vi "Menu.vi"() -> ()   [LabVIEW 2016]
uses:
  controls/Enum.ctl
  Course Project/support/Message Queue/Message Cluster.ctl
  <vilib>/FPGAPlugInAG/USB-7856R OEM/niLvFpga_Close_USB-7856R OEM.vi
  <vilib>/FPGAPlugInAG/USB-7856R OEM/niLvFpga_Reset_USB-7856R OEM.vi
  <vilib>/rvi/errors/niLvFpgaAdjustHostInterfaceError.vi
  <vilib>/rvi/interface/nirviCloseFPGA/nirviCloseFPGA.xnode
  controls/FPGAVIreferenceTypeDefScanEngine.ctl
  FPGA Bitfiles/qnmController797_usbRIO_controllerFPGAmu.lvbitx
  controls/FPGAVIreferenceTypeDef.ctl
  <vilib>/rvi/interface/nirviMethod/nirviMethod.xnode
  <vilib>/rvi/interface/nirviReadWriteControl/nirviReadWriteControl.xnode
  Course Project/support/Message Queue/Message Queue.lvlib
  Course Project/support/User Event - Stop/User Event - Stop.lvlib
  <vilib>/Utility/config.llb/NI_LVConfig.lvlib
  <vilib>/Utility/config.llb/Read Key (String).vi
  NiFpgaLv.dll
  controls/EnumSM.ctl
panel:
  in  "Clock":u32=1000000 format="%#_7pHz"
  in  "Custom ADC / DAC":bool
  out "Version":string="Version 02.08.2018"
  in  "Layout":enum32{"1", "2", "3", "4"}(radio)
  in  "Session path":path=path "C:/"
  in  "Create a new module":bool
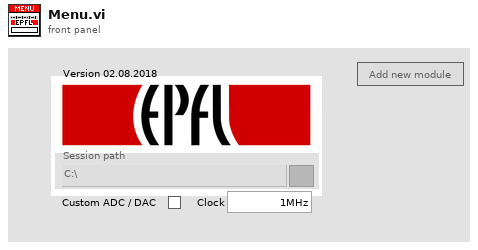
[diagram p1: front panel]
types:
  T1 = typedef "Message Queue.lvlib/All Message Queues.ctl" = cluster{"IU":refnum<queue>}
  T2 = typedef "Enum.ctl" = enum16{"Init", "Read", "Write"}
  T3 = typedef "EnumSM.ctl" = enum16{"Init.Calibrations", "Init.Excitation", "Init.StepMotor", "Init.FeedbackMotion", "Init.Scan", "Init.Signals", "Init.System", "Init.Waveform", "Init.ZController", "Send.Waveform", "Correct.Hysteresis"}
  T4 = enum32{"Bad", "Idle", "Run top level", "Running"}
  T5 = typedef "Message Queue.lvlib/Message Cluster.ctl" = cluster{"Message":string, "Données de message":variant}
  T6 = enum32{"Invalid", "Standard", "Closed", "Hidden", "Minimized", "Maximized"}
  T7 = enum16{"open", "replace", "create", "open or create", "replace or create", "replace or create with confirmation"}
  T8 = typedef "FPGAVIreferenceTypeDef.ctl" = refnum<k20>
  T9 = typedef "FPGAVIreferenceTypeDefScanEngine.ctl" = refnum<k20>
  T10 = typedef "NI_LVConfig.lvlib/Config Data RefNum.ctl" = refnum<k1>
  T11 = enum32{"Invalid", "Standard", "Closed", "Hidden", "Minimized", "Maximized"}[][]
  T12 = cluster{"offset past number":i32, "offset past number":i32}
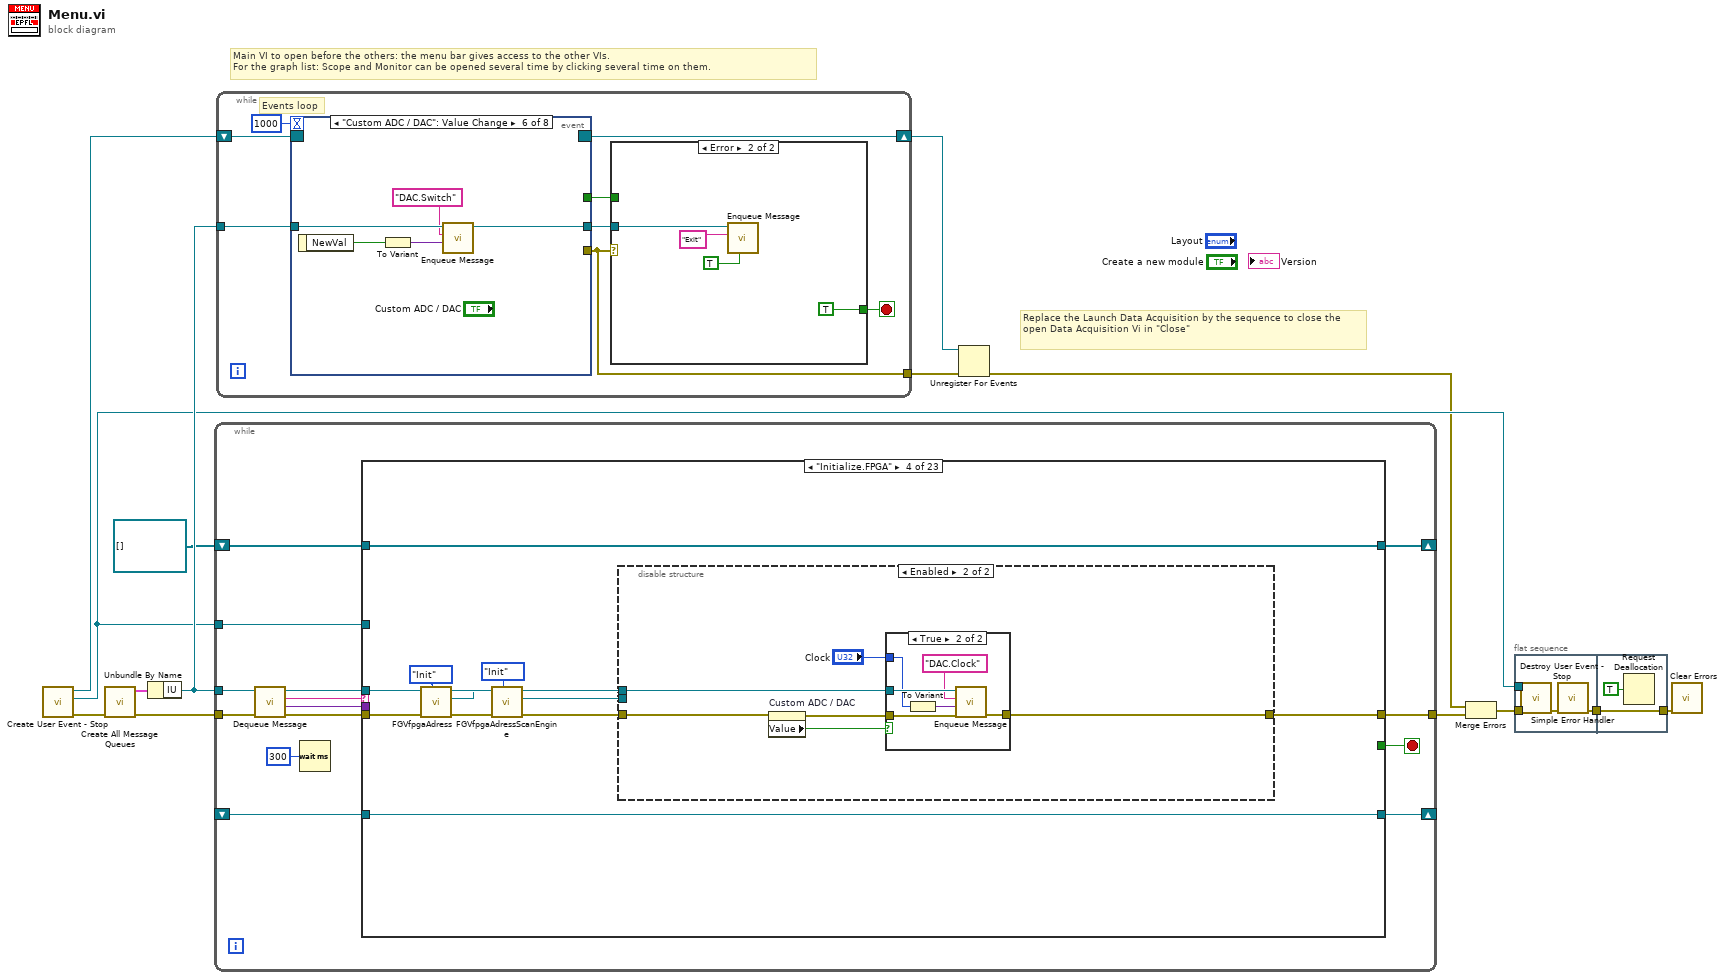
[diagram p0: block diagram]
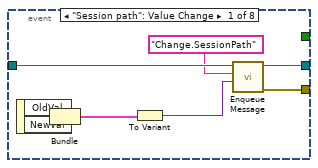
[diagram p3: hidden frame]
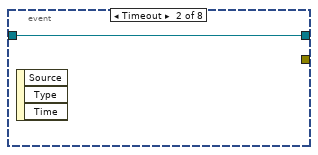
[diagram p4: hidden frame]
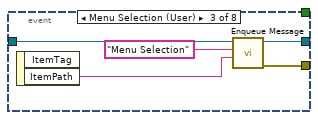
[diagram p5: hidden frame]
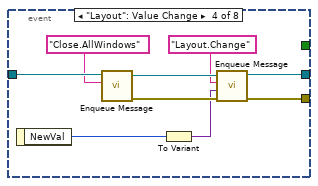
[diagram p6: hidden frame]
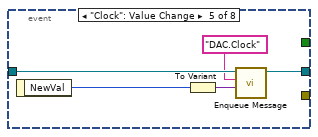
[diagram p7: hidden frame]
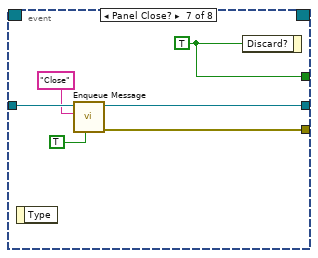
[diagram p8: hidden frame]
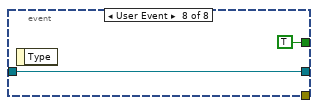
[diagram p9: hidden frame]
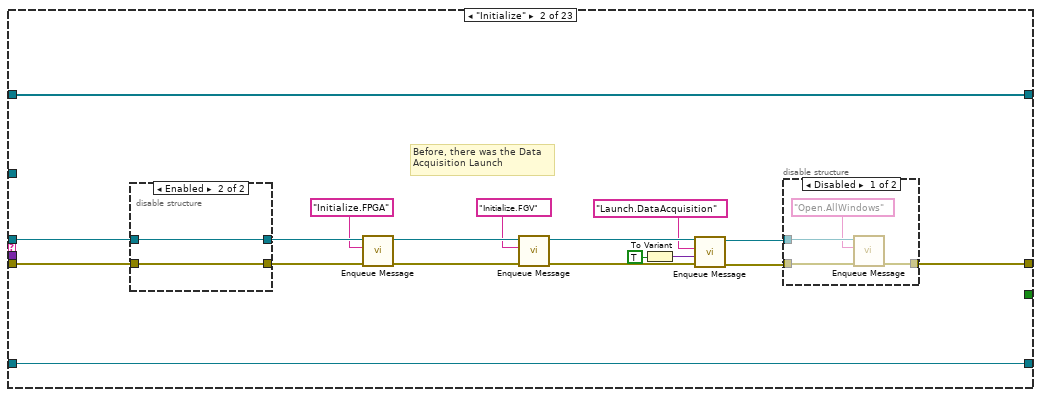
[diagram p11: hidden frame]
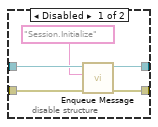
[diagram p12: hidden frame]
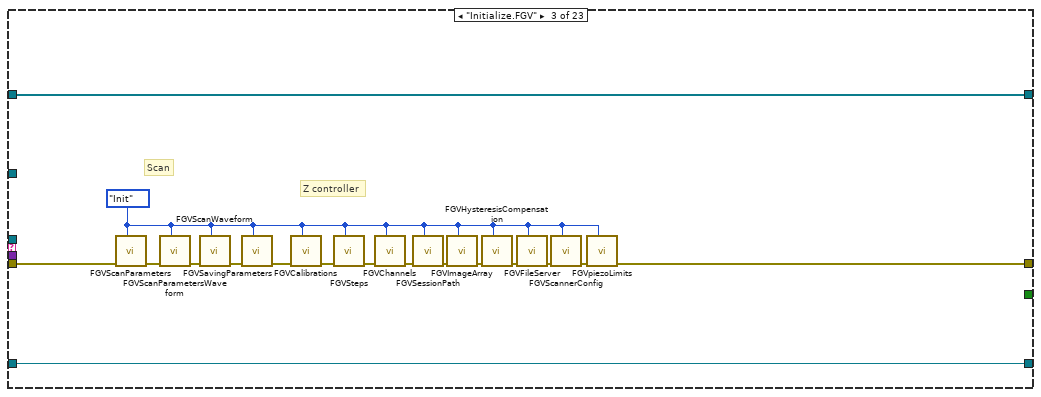
[diagram p14: hidden frame]
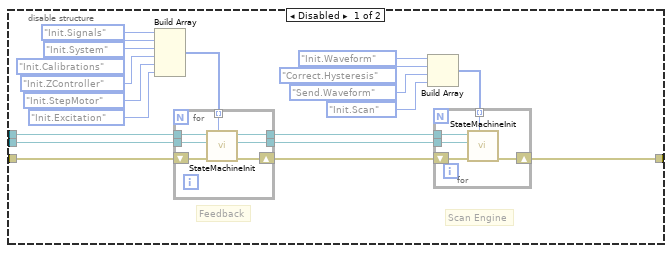
[diagram p15: hidden frame]
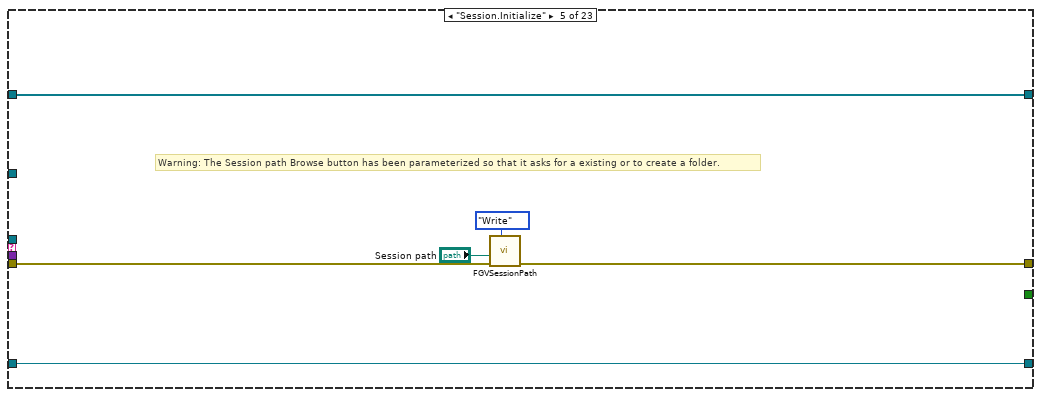
[diagram p17: hidden frame]
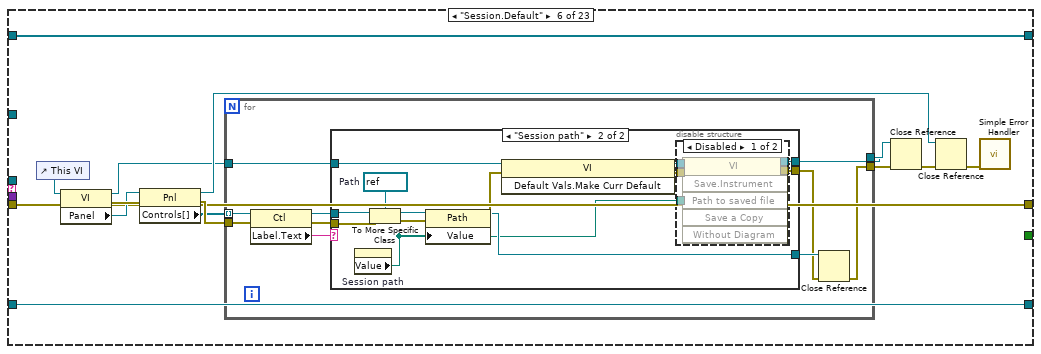
[diagram p18: hidden frame]
diagram:
  # "Main VI to open before the others: the menu bar gives access to the other VIs.\nFor the graph list: Scope and Monitor can be opened several time by clicking several time on them."
  # "Replace the Launch Data Acquisition by the sequence to close the open Data Acquisition Vi in \"Close\""
  n1 = call "Create User Event - Stop.vi"() -> ("sortie d'erreur"=w9:errorcluster, "Événement utilisateur - Arrêt"=w7:refnum<user-event>, "Refnum Enregistrement à l'événement Arrêt"=w10:refnum<event-registration>)  [unwired: 9 in]
  n2 = call "Create All Message Queues.vi"("ErrorIn"=w9) -> ("ErrorOut"=w14:errorcluster, "MessageQueueOut"=w13:T1)  [unwired: 9 in]
  n3 = Unbundle By Name(w13) -> ("IU"=w11:refnum<queue>)
  n4 = while {
    tunnel: w11 -> [w20]
    tunnel: w7 -> [w26]
    tunnel: w14 -> [w25]
    tunnel: [w27] -> w12
    shift-right: [w18] -> _
    shift-left: refnum<vi>[] [] -> [w17]
    shift-right: [w16] -> _
    shift-left: _ -> [w15]
    stop <- w28 stop-if-true
    n5 = call "Dequeue Message.vi"("entrée d'erreur (pas d'erreur)"=w25, "File d'attente de messages"=w20) -> ("sortie d'erreur"=w24:errorcluster, "Données de message"=w22:variant, "Message"=w23:string, "File d'attente de message dup."=w21:refnum<queue>)  [unwired: 6 in]
    n6 = Wait (ms)(milliseconds to wait=u32 300) -> ()  [unwired: 1 out]
    n7 = case "Conditions des messages" shown="\"Initialize.FPGA\"" w23 {
      selector: w23 -> [_ _ _ _ _ _ _ _ _ _ _ _ _ _ _ _ _ _ _ _ _ _ w637]
      tunnel: w21 -> [_ w47 _ w89 _ _ _ _ _ _ _ _ _ _ _ _ _ _ w544 w565 _ w623 _]
      tunnel: w24 -> [w31 w41 w70 w88 w136 w140 w192 w196 w248 w285 w311 w317 w378 w387 w393 w413 w436 w477 w542 w554 w580 w620 _]
      tunnel: [w31 w46 w63 w83 w135 w140 w192 w197 w252 w283 w311 w320 w377 w387 w390 errorcluster {"status"=FALSE, "code"=0, "source"=""} ("error out") w437 w473 w529 w555 w577 w601 w635] -> w27
      tunnel: [_ _ _ _ _ _ _ _ _ _ _ _ _ _ _ _ _ _ _ _ _ TRUE _] -> w28
      tunnel: w22 -> [_ _ _ _ _ _ _ w195 w246 w284 _ _ _ _ _ w412 w434 w476 w541 _ _ _ _]
      tunnel: w26 -> [_ _ _ _ _ _ _ _ _ _ _ _ _ _ _ _ _ _ _ _ _ w619 _]
      tunnel: [w30 w44 w78 w87 w139 w141 w189 w207 w254 w287 w309 w315 refnum<vi>[] [] w386 w391 w404 w431 w465 w531 w558 w594 w617 w633] -> w18
      tunnel: w17 -> [w30 w44 w78 w87 w139 w141 w189 w207 w254 w287 w309 _ w376 w386 w392 w404 w431 w465 w531 w558 w594 w617 w633]
      tunnel: [w29 w43 w77 w86 w138 w142 w187 w206 w253 w286 w310 w312 w374 w385 w389 w403 w430 w464 w530 w557 w593 w616 w632] -> w16
      tunnel: w15 -> [w29 w43 w77 w86 w138 w142 _ w206 w253 w286 w310 w314 w374 w385 w389 w403 w430 w464 w530 w557 w593 w616 w632]
      frame " ------- Init -------" {
      }
      frame "Initialize" {
        # "Before, there was the Data \nAcquisition Launch"
        n8 = disable-structure shown="Enabled" {
          disable-tunnel: [w54 w56] -> w48
          disable-tunnel: w47 -> [w53 w56]
          disable-tunnel: [w51 w55] -> w42
          disable-tunnel: w41 -> [w50 w55]
          frame Disabled {
            n9 = call "Enqueue Message.vi"("error in"=w50, "Message"="Session.Initialize", "Queue"=w53) -> ("error out"=w51:errorcluster, "Queue dup."=w54:refnum<queue>)  [unwired: 7 in]
          }
          frame Enabled {
          }
        }
        n10 = call "Enqueue Message.vi"("error in"=w42, "Message"="Initialize.FPGA", "Queue"=w48) -> ("error out"=w39:errorcluster, "Queue dup."=w40:refnum<queue>)  [unwired: 7 in]
        n11 = call "Enqueue Message.vi"("error in"=w39, "Message"="Initialize.FGV", "Queue"=w40) -> ("error out"=w35:errorcluster, "Queue dup."=w49:refnum<queue>)  [unwired: 7 in]
        n12 = To Variant(anything=TRUE) -> (Variant=w32:variant)
        n13 = call "Enqueue Message.vi"("error in"=w35, "Data"=w32, "Message"="Launch.DataAcquisition", "Queue"=w49) -> ("error out"=w36:errorcluster, "Queue dup."=w34:refnum<queue>)  [unwired: 6 in]
        n14 = disable-structure shown="Disabled" {
          disable-tunnel: w34 -> [w60 _]
          disable-tunnel: [w59 w61] -> w46
          disable-tunnel: w36 -> [w57 w61]
          frame Disabled {
            n15 = call "Enqueue Message.vi"("error in"=w57, "Message"="Open.AllWindows", "Queue"=w60) -> ("error out"=w59:errorcluster)  [unwired: 7 in, 1 out]
          }
          frame Enabled {
          }
        }
      }
      frame "Initialize.FGV" {
        w62 = Enum."Init" ("Enum")
        # "Z controller"
        # "Scan"
        n16 = call "FGVScanParameters.vi"("Enum"=w62, "error in"=w70) -> ("error out"=w76:errorcluster)  [unwired: 8 in, 1 out]
        n17 = call "FGVScanParametersWaveform.vi"("Enum"=w62, "error in"=w76) -> ("error out"=w75:errorcluster)  [unwired: 8 in, 1 out]
        n18 = call "FGVScanWaveform.vi"("Enum"=w62, "error in"=w75) -> ("error out"=w74:errorcluster)  [unwired: 8 in, 1 out]
        n19 = call "FGVSavingParameters.vi"("Enum"=w62, "error in"=w74) -> ("error out"=w73:errorcluster)  [unwired: 6 in, 3 out]
        n20 = call "FGVCalibrations.vi"("Enum"=w62, "error in"=w73) -> ("error out"=w72:errorcluster)  [unwired: 8 in, 1 out]
        n21 = call "FGVSteps.vi"("Enum"=w62, "error in"=w72) -> ("error out"=w71:errorcluster)  [unwired: 6 in, 3 out]
        n22 = call "FGVChannels.vi"("Enum"=w62, "error in"=w71) -> ("error out"=w69:errorcluster)  [unwired: 5 in, 4 out]
        n23 = call "FGVSessionPath.vi"("Enum"=w62, "error in"=w69) -> ("error out"=w68:errorcluster)  [unwired: 8 in, 1 out]
        n24 = call "FGVImageArray.vi"("Enum"=w62, "error in"=w68) -> ("error out"=w67:errorcluster)  [unwired: 8 in, 1 out]
        n25 = call "FGVHysteresisCompensation.vi"("Enum"=w62, "error in"=w67) -> ("error out"=w66:errorcluster)  [unwired: 7 in, 2 out]
        n26 = call "FGVFileServer.vi"("Enum"=w62, "error in"=w66) -> ("error out"=w65:errorcluster)  [unwired: 8 in, 1 out]
        n27 = call "FGVScannerConfig.vi"("Enum"=w62, "error in"=w65) -> ("error out"=w64:errorcluster)  [unwired: 7 in, 2 out]
        n28 = call "FGVpiezoLimits.vi"("Enum"=w62, "error in"=w64) -> ("error out"=w63:errorcluster)  [unwired: 8 in, 1 out]
      }
      frame "Initialize.FPGA" {
        n29 = call "FGVfpgaAdress.vi"("Enum"=Enum."Init", "error in"=w88) -> ("error out"=w80:errorcluster, "FPGA VI Reference Out"=w84:T8)  [unwired: 4 in, 4 out]
        n30 = call "FGVfpgaAdressScanEngine.vi"("Enum"=Enum."Init", "error in"=w80) -> ("error out"=w85:errorcluster, "FPGA.SEout"=w82:T9)  [unwired: 5 in, 3 out]
        n31 = disable-structure shown="Enabled" {
          disable-tunnel: w85 -> [w108 w126]
          disable-tunnel: w84 -> [w107 _]
          disable-tunnel: [w104 w124] -> w83
          disable-tunnel: w82 -> [w95 _]
          disable-tunnel: w89 -> [_ w122]
          frame Disabled {
            # "Feedback"
            # "Scan Engine"
            n32 = Build Array(EnumSM."Init.Signals" ("Enum"), EnumSM."Init.System" ("Enum"), EnumSM."Init.Calibrations" ("Enum"), EnumSM."Init.ZController" ("Enum"), EnumSM."Init.StepMotor" ("Enum"), EnumSM."Init.Excitation" ("Enum")) -> (w93:T3[])
            n33 = for {
              tunnel: w95 -> [w111]
              shift-right: [w112] -> w105
              shift-left: w108 -> [w115]
              tunnel: w93 -> [w110] mode=indexing
              tunnel: [w109] -> w92
              tunnel: w107 -> [w114]
              tunnel: [w113] -> w106
              n34 = call "StateMachineInit.vi"("Enum"=w110, "Error In"=w115, "FPGA.SEin"=w111, "FPGA.FBin"=w114) -> ("error out"=w112:errorcluster, "FPGA.SEout"=w109:T9, "FPGA.FBout"=w113:T8)  [unwired: 5 in]
            }
            n35 = Build Array(EnumSM."Init.Waveform" ("Enum"), EnumSM."Correct.Hysteresis" ("Enum"), EnumSM."Send.Waveform" ("Enum"), EnumSM."Init.Scan" ("Enum")) -> (w94:T3[])
            n36 = for {
              tunnel: w106 -> [w120]
              shift-right: [w118] -> w104
              shift-left: w105 -> [w119]
              tunnel: w94 -> [w117] mode=indexing
              tunnel: w92 -> [w116]
              n37 = call "StateMachineInit.vi"("Enum"=w117, "Error In"=w119, "FPGA.SEin"=w116, "FPGA.FBin"=w120) -> ("error out"=w118:errorcluster)  [unwired: 5 in, 2 out]
            }
          }
          frame Enabled {
            n38 = property on="Custom ADC / DAC" class="Bool (strict)"(error in=w126) -> (error out=w123:errorcluster, "Value"=w125:bool)  [unwired: 1 in, 1 out]
            n39 = case shown="True" w125 {
              tunnel: w122 -> [_ w133]
              tunnel: "Clock" -> [_ w132]
              tunnel: [w127 w129] -> w124
              tunnel: w123 -> [w127 w128]
              frame False {
              }
              frame True {
                n40 = To Variant(anything=w132) -> (Variant=w130:variant)
                n41 = call "Enqueue Message.vi"("error in"=w128, "Data"=w130, "Message"="DAC.Clock", "Queue"=w133) -> ("error out"=w129:errorcluster)  [unwired: 6 in, 1 out]
              }
            }
          }
        }
      }
      frame "Session.Initialize" {
        # "Warning: The Session path Browse button has been parameterized so that it asks for a existing or to create a folder."
        n42 = call "FGVSessionPath.vi"("Enum"=Enum."Write", "error in"=w136, "sessionPathIn"="Session path") -> ("error out"=w135:errorcluster)  [unwired: 7 in, 1 out]
      }
      frame "Session.Default" {
        n43 = control-ref of="This VI"() -> (w143:refnum<vi>)
        n44 = property on="Property Node" class="VI"(reference=w143) -> (reference out=w146:refnum<vi>, error out=w147:errorcluster, "Panel"=w144:refnum<vi>)  [unwired: 1 in]
        n45 = property on="Property Node" class="Pnl"(reference=w144, error in=w147) -> (reference out=w153:refnum<vi>, error out=w148:errorcluster, "Controls[]"=w145:refnum<vi>[])
        n46 = for {
          tunnel: w145 -> [w162] mode=indexing
          tunnel: w146 -> [w163]
          tunnel: w148 -> [w159]
          tunnel: [w154] -> w149
          tunnel: [w157] -> w150
          n47 = property on="Property Node" class="Ctl"(reference=w162, error in=w159) -> (reference out=w160:refnum<vi>, error out=w158:errorcluster, "Label.Text"=w161:string)
          n48 = case shown="\"Session path\"" w161 {
            tunnel: w163 -> [w165 w179]
            tunnel: w160 -> [w164 w174]
            tunnel: w158 -> [w166 w173]
            tunnel: [w166 w171] -> w155
            tunnel: [w165 w170] -> w157
            tunnel: [w164 w168] -> w156
            frame Default {
            }
            frame "Session path" {
              w176 = refnum<vi> refnum  # Path
              n49 = property on="Session path" class="Path"() -> ("Value"=w167:path)  [unwired: 2 in, 2 out]
              n50 = To More Specific Class(target class=w176, reference=w174, error in=w173) -> (specific class reference=w175:refnum<vi>, error out=w172:errorcluster)
              n51 = property on="Property Node" class="Path"(reference=w175, error in=w172, "Value"=w167) -> (reference out=w168:refnum<vi>, error out=w169:errorcluster)
              n52 = invoke class="VI" method="Default Vals.Make Curr Default"(reference=w179, error in=w169) -> (reference out=w178:refnum<vi>, error out=w177:errorcluster)  [unwired: 1 in, 1 out]
              n53 = disable-structure shown="Disabled" {
                disable-tunnel: w178 -> [w184 w186]
                disable-tunnel: w177 -> [w183 w185]
                disable-tunnel: [w182 w185] -> w171
                disable-tunnel: [w181 w186] -> w170
                disable-tunnel: w167 -> [w180 _]
                frame Disabled {
                  n54 = invoke class="VI" method="Save.Instrument"(reference=w184, error in=w183, "Path to saved file"=w180) -> (reference out=w181:refnum<vi>, error out=w182:errorcluster)  [unwired: 3 in, 4 out]
                }
                frame Enabled {
                }
              }
            }
          }
          n55 = Close Reference(reference=w156, error in (no error)=w155) -> (error out=w154:errorcluster)
        }
        n56 = Close Reference(reference=w150, error in (no error)=w149) -> (error out=w152:errorcluster)
        n57 = Close Reference(reference=w153, error in (no error)=w152) -> (error out=w151:errorcluster)
        n58 = call <vilib>:"Simple Error Handler.vi"("error in (no error)"=w151) -> ()  [unwired: 4 in, 5 out]
      }
      frame "Load.ConfigurationFile" {
        n59 = local read "Session path"() -> (w190:path)
        n60 = Build Path(base path=w190, name or relative path=path "ConfigurationFile.ini" ("default name")) -> (appended path=w188:path)
        n61 = call <vilib>:"Open Config Data.vi"("configuration file path"=w188) -> ("refnum"=w187:T10)  [unwired: 2 in, 8 out]
      }
      frame "Launch.DataAcquisition" {
        n62 = Variant To Data(error in=w196, type=TRUE, Variant=w195) -> (data=w205:bool, error out=w193:errorcluster)
        n63 = call <vilib>:"Application Directory.vi"() -> ("Application Directory"=w202:path)
        n64 = Build Path(base path=w202, name or relative path="FrontPanel\\subVIs\\DataAcquisition.vi") -> (appended path=w201:path)
        n65 = Open VI Reference(vi path=w201, error in (no error)=w193) -> (vi reference=w204:refnum<vi>, error out=w200:errorcluster)  [unwired: 4 in]
        n66 = case "Check the state of the VI: running or closed" shown="True" w205 {
          tunnel: w200 -> [w218 w228]
          tunnel: w204 -> [w211 w236]
          tunnel: [w208 w226] -> w198
          frame False {
            n67 = property class="VI"(reference=w211) -> (reference out=w219:refnum<vi>, "Exec.State"=w213:T4)  [unwired: 1 in, 1 out]
            n68 = Equal?(x=T4."Bad" ("Execution:State"), y=w213) -> (x = y?=w215:bool)
            n69 = Equal?(x=w213, y=T4."Idle" ("Execution:State")) -> (x = y?=w216:bool)
            n70 = Or(x=w215, y=w216) -> (x .or. y?=w217:bool)
            n71 = case shown="False" w217 {
              tunnel: [w223 w225] -> w210
              tunnel: [w222 w224] -> w209
              tunnel: w218 -> [w221 w224]
              tunnel: w219 -> [w220 w225]
              frame False {
                n72 = invoke class="VI" method="Abort VI"(reference=w220, error in=w221) -> (reference out=w223:refnum<vi>, error out=w222:errorcluster)  [unwired: 1 in, 1 out]
              }
              frame True {
              }
            }
            n73 = Close Reference(reference=w210, error in (no error)=w209) -> (error out=w208:errorcluster)
          }
          frame True {
            n74 = property class="VI"(reference=w236, error in=w228) -> (reference out=w235:refnum<vi>, error out=w227:errorcluster, "Exec.State"=w233:T4)
            n75 = Equal?(x=T4."Run top level" ("Execution:State"), y=w233) -> (x = y?=w231:bool)
            n76 = Equal?(x=w233, y=T4."Running" ("Execution:State")) -> (x = y?=w230:bool)
            n77 = Or(x=w231, y=w230) -> (x .or. y?=w229:bool)
            n78 = case shown="False" w229 {
              tunnel: [w238 w243] -> _
              tunnel: [w237 w242] -> w226
              tunnel: w227 -> [w239 w242]
              tunnel: w235 -> [w240 w243]
              frame False {
                n79 = invoke class="VI" method="Run VI"(reference=w240, error in=w239, "Wait until done"=FALSE ("Wait Until Done")) -> (reference out=w238:refnum<vi>, error out=w237:errorcluster)  [unwired: 2 in, 3 out]
              }
              frame True {
              }
            }
          }
        }
        n80 = call "FGVImageArray.vi"("Enum"=Enum."Init", "error in"=w198) -> ("error out"=w197:errorcluster)  [unwired: 8 in, 1 out]
      }
      frame "DAC.Switch" {
        n81 = Variant To Data(error in=w248, type=TRUE, Variant=w246) -> (data=w244:bool, error out=w247:errorcluster)
        n82 = call "FGVfpgaAdress.vi"("Enum"=Enum."Read", "error in"=w247) -> ("error out"=w250:errorcluster, "FPGA VI Reference Out"=w249:T8)  [unwired: 4 in, 4 out]
        n83 = xnode "Read/Write Control"("FPGA VI Reference In"=w249, "error in"=w250, "aio.o.fastInput"=w244) -> ("error out"=w252:errorcluster)  [unwired: 1 out]
      }
      frame "DAC.Clock" {
        w260 = 2.0 ("y")
        # "4 for 80MHz\n1 for 1Mhz"
        # "2 for the usb rio"
        n84 = Variant To Data(error in=w285, type=u32 0 ("NewVal"), Variant=w284) -> (data=w278:u32, error out=w288:errorcluster)
        n85 = call "FGVfpgaAdress.vi"("Enum"=Enum."Read", "error in"=w288) -> ("error out"=w276:errorcluster, "baseClockOut"=w256:u32, "FPGA VI Reference Out"=w273:T8, "voltageRange(+/-)Out"=w274:dbl)  [unwired: 4 in, 2 out]
        n86 = Multiply(x=w256, y=u32 1 ("x")) -> (x*y=w257:u32)
        n87 = Divide(x=w257, y=w278) -> (x/y=w272:dbl)
        n88 = Divide(x=w272, y=w260) -> (x/y=w269:dbl)
        n89 = To Unsigned Word Integer(number=w269) -> (unsigned 16bit integer=w261:u16)
        n90 = xnode "Read/Write Control"("FPGA VI Reference In"=w273, "error in"=w276, "aio.p.fastADCclockdec"=w261) -> ("FPGA VI Reference Out"=w271:T8, "error out"=w277:errorcluster)
        n91 = Divide(x=w257, y=w261) -> (x/y=w259:dbl)
        n92 = Divide(x=w259, y=w260) -> (x/y=w258:dbl)
        n93 = To Unsigned Long Integer(number=w258) -> (unsigned 32bit integer=w264:u32)
        n94 = call "FGVfpgaAdress.vi"("ioFreqHzIn"=w264, "Enum"=Enum."Write", "error in"=w277, "BaseClockIn"=w256, "FPGA VI Reference In"=w271, "voltageRange(+/-)In"=w274) -> ("error out"=w263:errorcluster)  [unwired: 5 out]
        n95 = property on="Clock" class="DigNum (strict)"(error in=w263, "Value"=w264) -> (error out=w262:errorcluster)  [unwired: 1 in, 1 out]
        n96 = call "IsVIRunning.vi"("error in (no error)"=w262, "name or relative path"="FrontPanel\\Excitation.vi") -> ("error out"=w267:errorcluster, "RunningVI?"=w266:bool)  [unwired: 8 in]
        n97 = disable-structure shown="Enabled" {
          disable-tunnel: [w291 w300] -> w268
          disable-tunnel: w267 -> [w290 w300]
          disable-tunnel: w266 -> [w289 _]
          frame Enabled {
            n98 = case shown="True" w289 {
              tunnel: [w292 w298] -> w291
              tunnel: w290 -> [w292 w294]
              frame False {
              }
              frame True {
                n99 = Obtain Queue(name (unnamed)="Excitation" ("QueueName"), element data type=T5 {"Message"="", "Données de message"=variant} ("Cluster Message"), error in (no error)=w294) -> (queue out=w299:refnum<queue>, error out=w293:errorcluster)  [unwired: 2 in, 1 out]
                n100 = call "Enqueue Message.vi"("error in"=w293, "Message"="Menu.ChangeClock", "Queue"=w299) -> ("error out"=w298:errorcluster)  [unwired: 7 in, 1 out]
              }
            }
          }
          frame Disabled {
          }
        }
        n101 = call "IsVIRunning.vi"("error in (no error)"=w268, "name or relative path"="FrontPanel\\ZController.vi") -> ("error out"=w281:errorcluster, "RunningVI?"=w280:bool)  [unwired: 8 in]
        n102 = case shown="True" w280 {
          tunnel: [w301 w307] -> w283
          tunnel: w281 -> [w301 w303]
          frame False {
          }
          frame True {
            n103 = Obtain Queue(name (unnamed)="ZController" ("QueueName"), element data type=T5 {"Message"="", "Données de message"=variant} ("Cluster Message"), error in (no error)=w303) -> (queue out=w308:refnum<queue>, error out=w302:errorcluster)  [unwired: 2 in, 1 out]
            n104 = call "Enqueue Message.vi"("error in"=w302, "Message"="Controllers.IOFrequency", "Queue"=w308) -> ("error out"=w307:errorcluster)  [unwired: 7 in, 1 out]
          }
        }
      }
      frame "------- Windows -------" {
      }
      frame "Open.AllWindows" {
        w313 = "WindowPositions"  # Section
        w316 = T11 [[enum."Standard", enum."Standard", enum."Standard", enum."Standard"], [enum."Standard", enum."Standard", enum."Hidden", enum."Standard"], [enum."Standard", enum."Standard", enum."Standard", enum."Standard"], [enum."Standard", enum."Standard", enum."Hidden", enum."Standard"], [enum."Standard", enum."Hidden", enum."Standard", enum."Hidden"], [enum."Closed", enum."Standard", enum."Standard", enum."Hidden"], [enum."Closed", enum."Hidden", enum."Standard", enum."Standard"], [enum."Closed", enum."Closed", enum."Closed", enum."Closed"]] items=["Invalid", "Standard", "Closed", "Hidden", "Minimized", "Maximized"]
        # "Take the names from the menu.rtm"
        # "Add window position from configuration file"
        # "4"
        # "3"
        # "2"
        # "Layout"
        # "1"
        # "Windows config for layouts"
        n105 = for {
          tunnel: "Monitor" -> [w343]
          tunnel: string[] ["Calibration", "Signals", "Scan", "ZController", "Monitor", "3xMonitor", "4xMonitor", "Waveforms"] -> [w327] mode=indexing
          tunnel: w316 -> [w334]
          tunnel: w317 -> [_]
          tunnel: [w330] -> w320
          tunnel: [w329] -> w315 mode=indexing
          tunnel: w314 -> [w324]
          tunnel: w313 -> [w323]
          tunnel: [w322] -> w312
          i -> [w333]
          n106 = Not Equal?(x=w327, y=w343) -> (x != y?=w335:bool)
          n107 = Select(t=".vi", s=w335, f=".vit") -> (s? t:f=w326:string)
          n108 = local read "Layout"() -> (w332:enum32{"1", "2", "3", "4"})
          n109 = call <vilib>:"Application Directory.vi"() -> ("Application Directory"=w339:path)
          n110 = Concatenate Strings("FrontPanel\\" ("string"), w327, w326) -> (w342:string)
          n111 = Concatenate Strings(w327, w326) -> (w325:string)
          n112 = Build Path(base path=w339, name or relative path=w342) -> (appended path=w341:path)
          n113 = Index Array(array=w334, index (row)=w333, index (col)=w332) -> (element=w331:T6)
          n114 = Open VI Reference(vi path=w341) -> (vi reference=w338:refnum<vi>, error out=w321:errorcluster)  [unwired: 5 in]
          n115 = case shown="No Error" w321 {
            selector: w321 -> [w344 w357]
            tunnel: w338 -> [w353 w358]
            tunnel: w331 -> [w352 _]
            tunnel: [w351 w357] -> w330
            tunnel: [w350 w358] -> w329
            tunnel: [w349 _] -> w328
            frame No Error {
              n116 = invoke class="VI" method="FP.Open"(reference=w353, error in=w344, "Activate"=TRUE ("Activate?"), "State"=w352) -> (reference out=w348:refnum<vi>, error out=w347:errorcluster)  [unwired: 1 in, 3 out]
              n117 = property class="VI"(reference=w348, error in=w347) -> (reference out=w346:refnum<vi>, error out=w345:errorcluster, "Panel"=w349:refnum<vi>)
              n118 = invoke class="VI" method="Run VI"(reference=w346, error in=w345, "Wait until done"=FALSE ("Wait Until Done"), "Auto Dispose Ref"=FALSE ("Auto Dispose Reference")) -> (reference out=w350:refnum<vi>, error out=w351:errorcluster)  [unwired: 1 in, 3 out]
            }
            frame Error {
            }
          }
          n119 = disable-structure shown="Disabled" {
            disable-tunnel: w328 -> [w372 _]
            disable-tunnel: w325 -> [w370 _]
            disable-tunnel: w324 -> [w369 w373]
            disable-tunnel: w323 -> [w368 _]
            disable-tunnel: [w367 w373] -> w322
            frame Disabled {
              n120 = call-poly <vilib>:"Read Key.vi"("section"=w368, "key"=w370, "refnum"=w369) -> ("value"=w366:string, "refnum out"=w367:T10)  [unwired: 5 in, 2 out]
              n121 = call <vilib>:"Space Constant.vi"() -> ("String"=w365:string)
              n122 = Match Pattern(string=w366, regular expression=w365) -> (before substring=w363:string, after substring=w362:string)  [unwired: 1 in, 2 out]
              n123 = call <vilib>:"Space Constant.vi"() -> ("String"=w364:string)
              n124 = Match Pattern(string=w362, regular expression=w364) -> (before substring=w359:string)  [unwired: 1 in, 3 out]
              n125 = Decimal String To Number(string=w363) -> (offset past number=w361:i32)  [unwired: 2 in, 1 out]
              n126 = Decimal String To Number(string=w359) -> (offset past number=w360:i32)  [unwired: 2 in, 1 out]
              n127 = Bundle("offset past number"=w361, "offset past number"=w360) -> (w371:T12)  [unwired: 1 in]
              n128 = property class="Pnl"(reference=w372, "Position"=w371) -> ()  [unwired: 1 in, 2 out]
            }
            frame Enabled {
            }
          }
        }
      }
      frame "Close.AllWindows" {
        n129 = for {
          tunnel: w378 -> [w380]
          tunnel: [w384] -> w377
          tunnel: w376 -> [w381] mode=indexing
          n130 = property class="VI"(reference=w381, error in=w380, "Front Panel Window:State"=T6."Closed") -> (reference out=w383:refnum<vi>, error out=w382:errorcluster)
          n131 = Close Reference(reference=w383, error in (no error)=w382) -> (error out=w384:errorcluster)
        }
      }
      frame "------- Layouts -------" {
      }
      frame "Layout.Change" {
        w394 = T11 [[enum."Standard", enum."Standard", enum."Standard", enum."Standard"], [enum."Standard", enum."Standard", enum."Hidden", enum."Hidden"], [enum."Hidden", enum."Hidden", enum."Standard", enum."Hidden"], [enum."Hidden", enum."Hidden", enum."Hidden", enum."Standard"], [enum."Closed", enum."Closed", enum."Closed", enum."Closed"], [enum."Closed", enum."Closed", enum."Closed", enum."Closed"], [enum."Closed", enum."Closed", enum."Closed", enum."Closed"], [enum."Closed", enum."Closed", enum."Closed", enum."Closed"]] items=["Invalid", "Standard", "Closed", "Hidden", "Minimized", "Maximized"]
        n132 = local read "Layout"() -> (w388:enum32{"1", "2", "3", "4"})
        n133 = for {
          tunnel: w394 -> [w402]
          tunnel: w393 -> [w400]
          tunnel: w392 -> [w398] mode=indexing
          tunnel: [w397] -> w391 mode=indexing
          tunnel: [w396] -> w390
          tunnel: w388 -> [w395]
          i -> [w401]
          n134 = Index Array(array=w402, index (row)=w401, index (col)=w395) -> (element=w399:T6)
          n135 = property class="VI"(reference=w398, error in=w400, "Front Panel Window:State"=w399) -> (reference out=w397:refnum<vi>, error out=w396:errorcluster)
        }
      }
      frame "Open Settings" {
        # "Replace when there will finally be a Settings.ini file"
        n136 = Variant To Data(error in=w413, type=path "", Variant=w412) -> (data=w407:path, error out=w410:errorcluster)
        n137 = call "FGVSessionPath.vi"("Enum"=Enum."Write", "error in"=w410, "sessionPathIn"=w407) -> ("error out"=w409:errorcluster, "sessionPathOut"=w406:path)  [unwired: 7 in]
        n138 = disable-structure shown="Disabled" {
          disable-tunnel: w409 -> [w416 _]
          disable-tunnel: w406 -> [w414 _]
          frame Disabled {
            (unwired) "Session.ini"
            # "Do the same for Session"
            n139 = Build Path(base path=w414, name or relative path="Settings.ini") -> (appended path=w422:path)
            n140 = Open/Create/Replace File(file path (use dialog)=w422, error in=w416, operation (0:open)=T7."replace or create") -> (refnum out=w419:refnum<file>, error out=w420:errorcluster)  [unwired: 3 in, 1 out]
            n141 = disable-structure shown="Disabled" {
              disable-tunnel: w420 -> [w427 w429]
              disable-tunnel: w419 -> [w426 w428]
              disable-tunnel: [w425 w429] -> w418
              disable-tunnel: [w424 w428] -> w417
              frame Disabled {
                n142 = Scan From String(w426, w427) -> (w424:refnum<file>, w425:errorcluster)  [unwired: 3 in]
                n143 = call "FGVScanParametersWaveform.vi"("Enum"=Enum."Read") -> ()  [unwired: 9 in, 2 out]
              }
              frame Enabled {
              }
            }
            n144 = Close File(refnum=w417, error in=w418) -> ()  [unwired: 2 out]
          }
          frame Enabled {
          }
        }
      }
      frame "Save Settings" {
        n145 = Variant To Data(error in=w436, type=path "", Variant=w434) -> (data=w432:path, error out=w435:errorcluster)
        n146 = Two Button Dialog(message="Save the current settings to the previous session folder?", 1:"No" ("T button name (\"OK\")"), 2:"Yes" ("T button name (\"OK\")")) -> (T button?=w438:bool)
        n147 = disable-structure shown="Disabled" {
          disable-tunnel: w438 -> [w445 _]
          disable-tunnel: [w444 w462] -> w437
          disable-tunnel: w435 -> [w443 w462]
          disable-tunnel: w432 -> [w442 _]
          frame Disabled {
            n148 = case shown="True" w445 {
              tunnel: w443 -> [w446 w454]
              tunnel: [w446 w453] -> w444
              tunnel: w442 -> [_ w452]
              frame False {
              }
              frame True {
                # "needs to read all parameters"
                # "replace the config file with the new settings"
                n149 = Open/Create/Replace File(file path (use dialog)=w452, error in=w454, operation (0:open)=T7."replace") -> (refnum out=w448:refnum<file>, error out=w450:errorcluster)  [unwired: 3 in, 1 out]
                n150 = disable-structure shown="Disabled" {
                  disable-tunnel: w450 -> [w459 w460]
                  disable-tunnel: [w458 w460] -> w449
                  disable-tunnel: w448 -> [w457 w461]
                  disable-tunnel: [w456 w461] -> w447
                  frame Disabled {
                    n151 = Format Into String(initial string=w457, error in=w459) -> (resulting string=w456:refnum<file>, error out=w458:errorcluster)  [unwired: 2 in]
                    n152 = call "FGVScanParametersWaveform.vi"("Enum"=Enum."Read") -> ()  [unwired: 9 in, 2 out]
                  }
                  frame Enabled {
                  }
                }
                n153 = Close File(refnum=w447, error in=w449) -> (error out=w453:errorcluster)  [unwired: 1 out]
              }
            }
          }
          frame Enabled {
          }
        }
      }
      frame "Menu Selection" {
        n154 = Variant To Data(error in=w477, type="", Variant=w476) -> (data=w468:string, error out=w474:errorcluster)
        n155 = Search/Split String(string=w468, search string/char (-)=":") -> (substring before match=w471:string, match + rest of string=w470:string)  [unwired: 1 in, 1 out]
        n156 = String Subset(string=w470, offset (0)=1) -> (substring=w467:string)  [unwired: 1 in]
        n157 = case shown="\"Experiments\", \"Graphs\", \"Modules\", \"System\"" w471 {
          tunnel: w474 -> [w479 w513]
          tunnel: [w479 w509] -> w473
          tunnel: w467 -> [w478 w514]
          tunnel: "Monitor" -> [_ w500]
          tunnel: "Scope" -> [_ w502]
          frame "File", Default {
            n158 = case shown="\"Abort\"" w478 {
              frame "False", Default {
              }
              frame "Abort" {
                # "/!\\ VIOLENT /!\\"
                n159 = flat-sequence {
                  frame #0 {
                    w488 = Enum."Read" ("Enum")
                    n160 = call "FGVfpgaAdress.vi"("Enum"=w488) -> ("error out"=w485:errorcluster, "FPGA VI Reference Out"=w486:T8)  [unwired: 5 in, 4 out]
                    n161 = call "FGVfpgaAdressScanEngine.vi"("Enum"=w488) -> ("error out"=w484:errorcluster, "FPGA.SEout"=w487:T9)  [unwired: 6 in, 3 out]
                    n162 = xnode "Invoke Method"("FPGA VI Reference In"=w486, "error in"=w485) -> ("FPGA VI Reference Out"=w483:T8, "error out"=w480:errorcluster)
                    n163 = xnode "Invoke Method"("FPGA VI Reference In"=w487, "error in"=w484) -> ("FPGA VI Reference Out"=w482:T9, "error out"=w481:errorcluster)
                    n164 = xnode "Close FPGA VI Reference"("FPGA VI Reference In"=w483, "error in"=w480) -> ()  [unwired: 1 out]
                    n165 = xnode "Close FPGA VI Reference"("FPGA VI Reference In"=w482, "error in"=w481) -> ()  [unwired: 1 out]
                  }
                  frame #1 {
                    n166 = Quit LabVIEW() -> ()  [unwired: 1 in]
                  }
                }
              }
            }
          }
          frame "Experiments", "Graphs", "Modules", "System" {
            n167 = Equal?(x=w514, y=w502) -> (x = y?=w501:bool)
            n168 = Equal?(x=w514, y=w500) -> (x = y?=w499:bool)
            n169 = Or(x=w499, y=w501) -> (x .or. y?=w498:bool)
            n170 = Select(t=".vit", s=w498, f=".vi") -> (s? t:f=w503:string)
            n171 = call <vilib>:"Application Directory.vi"() -> ("Application Directory"=w507:path)
            n172 = Concatenate Strings("FrontPanel\\" ("string"), w514, w503) -> (w512:string)
            n173 = Build Path(base path=w507, name or relative path=w512) -> (appended path=w511:path)
            n174 = Open VI Reference(vi path=w511, error in (no error)=w513) -> (vi reference=w506:refnum<vi>, error out=w510:errorcluster)  [unwired: 4 in]
            n175 = case shown="\"Monitor\", \"Scope\"" w514 {
              selector: w514 -> [w516 _]
              tunnel: w506 -> [w523 w526]
              tunnel: [w522 w524] -> w489
              tunnel: w510 -> [_ w525]
              frame "Monitor", "Scope" {
                n176 = feedback #1(1.0) -> (w518:dbl)
                n177 = Increment(x=w518) -> (x+1=w519:dbl)
                n178 = feedback-in #1(w519) -> ()
                n179 = Number To Decimal String(number=w518) -> (decimal integer string=w520:string)  [unwired: 1 in]
                n180 = Concatenate Strings(w516, " #" ("string"), w520) -> (w521:string)
                n181 = property class="VI"(reference=w523, "Front Panel.Title"=w521) -> (reference out=w522:refnum<vi>)  [unwired: 1 in, 1 out]
              }
              frame Default {
                # "remote"
                n182 = property class="VI" props=["Front Panel.Title"](reference=w526, error in=w525) -> (reference out=w524:refnum<vi>)  [unwired: 2 out]
              }
            }
            n183 = invoke class="VI" method="FP.Open"(reference=w489, error in=w510, "Activate"=TRUE ("Activate?"), "State"=T6."Standard") -> (reference out=w497:refnum<vi>, error out=w496:errorcluster)  [unwired: 1 in, 3 out]
            n184 = invoke class="VI" method="Run VI"(reference=w497, error in=w496, "Wait until done"=FALSE ("Wait Until Done"), "Auto Dispose Ref"=FALSE ("Auto Dispose Reference")) -> (reference out=w490:refnum<vi>, error out=w491:errorcluster)  [unwired: 1 in, 3 out]
            n185 = Close Reference(reference=w490, error in (no error)=w491) -> (error out=w509:errorcluster)
          }
        }
      }
      frame "Change.SessionPath" {
        # "When the session path is changed, a window should pop up to ask the user is he wants to save the previous settings/configuration to the previous session"
        n186 = Variant To Data(error in=w542, type=cluster{"OldVal":path, "NewVal":path} {"OldVal"=path "", "NewVal"=path ""} ("output cluster"), Variant=w541) -> (data=w539:cluster{"OldVal":path, "NewVal":path}, error out=w537:errorcluster)
        n187 = Unbundle By Name(w539) -> ("NewVal"=w533:path, "OldVal"=w538:path)
        n188 = To Variant(anything=w538) -> (Variant=w528:variant)
        n189 = To Variant(anything=w533) -> (Variant=w527:variant)
        n190 = call "Enqueue Message.vi"("error in"=w537, "Data"=w528, "Message"="Save Settings", "Queue"=w544) -> ("error out"=w536:errorcluster, "Queue dup."=w535:refnum<queue>)  [unwired: 6 in]
        n191 = call "Enqueue Message.vi"("error in"=w536, "Data"=w527, "Message"="Open Settings", "Queue"=w535) -> ("error out"=w532:errorcluster, "Queue dup."=w545:refnum<queue>)  [unwired: 6 in]
        n192 = disable-structure shown="Disabled" {
          disable-tunnel: w545 -> [w549 _]
          disable-tunnel: w532 -> [w547 w550]
          disable-tunnel: [w546 w550] -> w529
          frame Disabled {
            n193 = call "Enqueue Message.vi"("error in"=w547, "Message"="Update Settings", "Queue"=w549) -> ("error out"=w546:errorcluster)  [unwired: 7 in, 1 out]
          }
          frame Enabled {
          }
        }
      }
      frame "Close" {
        # "Close Data Acquisition"
        n194 = call "Enqueue Message.vi"("error in"=w554, "Message"="Session.Default", "Queue"=w565) -> ("error out"=w553:errorcluster, "Queue dup."=w564:refnum<queue>)  [unwired: 7 in]
        n195 = call "Enqueue Message.vi"("error in"=w553, "Data"=FALSE, "Message"="Launch.DataAcquisition", "Queue"=w564) -> ("error out"=w559:errorcluster, "Queue dup."=w563:refnum<queue>)  [unwired: 6 in]
        n196 = disable-structure shown="Enabled" {
          disable-tunnel: w563 -> [w571 w576]
          disable-tunnel: [w570 w574] -> w562
          disable-tunnel: [w568 w573] -> w560
          disable-tunnel: w559 -> [w567 w572]
          frame Disabled {
            n197 = call "Enqueue Message.vi"("error in"=w567, "Data"=FALSE ("Message prioritaire ? (F)"), "Message"="Close.AllWindows", "Queue"=w571) -> ("error out"=w568:errorcluster, "Queue dup."=w570:refnum<queue>)  [unwired: 6 in]
          }
          frame Enabled {
            n198 = call "Enqueue Message.vi"("error in"=w572, "Message"="Close.Calibration", "Queue"=w576) -> ("error out"=w573:errorcluster, "Queue dup."=w574:refnum<queue>)  [unwired: 7 in]
          }
        }
        n199 = call "Enqueue Message.vi"("error in"=w560, "Message"="Exit", "Queue"=w562) -> ("error out"=w555:errorcluster)  [unwired: 7 in, 1 out]
      }
      frame "Close.Calibration" {
        n200 = call <vilib>:"Application Directory.vi"() -> ("Application Directory"=w592:path)
        n201 = Build Path(base path=w592, name or relative path="FrontPanel\\Calibration.vi") -> (appended path=w590:path)
        n202 = Open VI Reference(vi path=w590, error in (no error)=w580) -> (vi reference=w581:refnum<vi>, error out=w582:errorcluster)  [unwired: 4 in]
        n203 = property class="VI"(reference=w581) -> (reference out=w589:refnum<vi>, "Exec.State"=w587:T4)  [unwired: 1 in, 1 out]
        n204 = Equal?(x=w587, y=T4."Running" ("Execution:State")) -> (x = y?=w584:bool)
        n205 = Equal?(x=T4."Run top level" ("Execution:State"), y=w587) -> (x = y?=w585:bool)
        n206 = Or(x=w585, y=w584) -> (x .or. y?=w583:bool)
        n207 = case shown="True" w583 {
          tunnel: [w596 w598] -> w579
          tunnel: [w595 w597] -> w578
          tunnel: w582 -> [w595 w599]
          tunnel: w589 -> [w596 w600]
          frame False {
          }
          frame True {
            n208 = invoke class="VI" method="Abort VI"(reference=w600, error in=w599) -> (reference out=w598:refnum<vi>, error out=w597:errorcluster)  [unwired: 1 in, 1 out]
          }
        }
        n209 = Close Reference(reference=w579, error in (no error)=w578) -> (error out=w577:errorcluster)
      }
      frame "Exit" {
        # "Open a window to propose the option of Stopping the scan and stopping DataAcquisition.vi"
        n210 = call "Fire User Event - Stop.vi"("Événement utilisateur - Arrêt"=w619) -> ("sortie d'erreur"=w618:errorcluster)  [unwired: 10 in]
        n211 = Release Queue(queue=w623, error in (no error)=w620) -> (error out=w621:errorcluster)  [unwired: 1 in, 2 out]
        n212 = Merge Errors(w618, w621) -> (w615:errorcluster)
        n213 = call "FGVImageArray.vi"("Enum"=Enum."Read", "error in"=w615) -> ("error out"=w602:errorcluster, "ImageRefOut"=w613:refnum<data-value>[][])  [unwired: 8 in]
        n214 = for {
          tunnel: w613 -> [w630] mode=indexing
          n215 = for {
            tunnel: w630 -> [w631] mode=indexing
            n216 = Delete Data Value Reference(data value reference=w631) -> ()  [unwired: 1 in, 2 out]
          }
        }
        n217 = call "FGVfpgaAdress.vi"("Enum"=Enum."Read", "error in"=w602) -> ("error out"=w604:errorcluster, "FPGA VI Reference Out"=w607:T8)  [unwired: 4 in, 4 out]
        n218 = disable-structure shown="Disabled" {
          disable-tunnel: w604 -> [w627 w629]
          disable-tunnel: [w626 w629] -> w605
          disable-tunnel: w607 -> [w625 w628]
          disable-tunnel: [w624 w628] -> w606
          frame Disabled {
            n219 = xnode "Invoke Method"("FPGA VI Reference In"=w625, "error in"=w627) -> ("FPGA VI Reference Out"=w624:T8, "error out"=w626:errorcluster)
          }
          frame Enabled {
          }
        }
        n220 = xnode "Close FPGA VI Reference"("FPGA VI Reference In"=w606, "error in"=w605) -> ("error out"=w608:errorcluster)
        n221 = call "FGVfpgaAdressScanEngine.vi"("Enum"=Enum."Read", "error in"=w608) -> ("error out"=w609:errorcluster, "FPGA.SEout"=w610:T9)  [unwired: 5 in, 3 out]
        n222 = xnode "Close FPGA VI Reference"("FPGA VI Reference In"=w610, "error in"=w609) -> ("error out"=w612:errorcluster)
        n223 = call <vilib>:"Simple Error Handler.vi"("error in (no error)"=w612) -> ("error out"=w601:errorcluster)  [unwired: 4 in, 4 out]
      }
      frame Default {
        n224 = Format Into String(format string="The message\"%s\" received in the gestion loop is not valid" ("Texte de message d'erreur inconnu"), w637) -> (resulting string=w634:string)  [unwired: 2 in, 1 out]
        n225 = call <vilib>:"Error Cluster From Error Code.vi"("error message (\"\")"=w634, "error code (0)"=1 ("code d'erreur (0)")) -> ("error out"=w635:errorcluster)  [unwired: 7 in]
      }
    }
  }
  n226 = while {
    tunnel: w11 -> [w646]
    tunnel: [w642] -> w6
    shift-right: [w640] -> w5
    shift-left: w10 -> [w641]
    stop <- w644 stop-if-true
    # "Events loop"
    n227 = event shown="[5] \"Custom ADC / DAC\": Value Change" {
      selector: w641 -> [_ _ _ _ _ _ _ _]
      dyn-events: [_ _ _ _ _ _ _ _] -> w640
      timeout: 1000 -> [_ _ _ _ _ _ _ _]
      tunnel: [_ _ _ _ _ _ w689 TRUE ("Rejeter ?")] -> w645
      tunnel: w646 -> [w659 w660 w665 w673 w679 w684 w688 w692]
      tunnel: [w658 _ w663 w667 _ _ w685 _] -> w642
      tunnel: [w657 w660 w664 w671 w678 w683 w686 w692] -> w643
      event "Session path": Value Change {
        n228 = event-data() -> ("OldVal"=w653:path, "NewVal"=w654:path)  [unwired: 1 in]
        n229 = Bundle("OldVal"=w653, "NewVal"=w654) -> (w652:cluster{"OldVal":path, "NewVal":path})  [unwired: 1 in]
        n230 = To Variant(anything=w652) -> (Variant=w655:variant)
        n231 = call "Enqueue Message.vi"("Data"=w655, "Message"="Change.SessionPath", "Queue"=w659) -> ("error out"=w658:errorcluster, "Queue dup."=w657:refnum<queue>)  [unwired: 7 in]
      }
      event Timeout {
        n232 = event-data() -> ()  [unwired: 1 in, 3 out]
      }
      event Menu Selection (User) {
        n233 = event-data() -> ("ItemPath"=w661:string)  [unwired: 1 in, 1 out]
        n234 = call "Enqueue Message.vi"("Data"=w661, "Message"="Menu Selection", "Queue"=w665) -> ("error out"=w663:errorcluster, "Queue dup."=w664:refnum<queue>)  [unwired: 7 in]
      }
      event "Layout": Value Change {
        n235 = event-data() -> ("NewVal"=w669:enum32{"1", "2", "3", "4"})  [unwired: 1 in]
        n236 = call "Enqueue Message.vi"("Message"="Close.AllWindows", "Queue"=w673) -> ("error out"=w668:errorcluster, "Queue dup."=w674:refnum<queue>)  [unwired: 8 in]
        n237 = To Variant(anything=w669) -> (Variant=w666:variant)
        n238 = call "Enqueue Message.vi"("error in"=w668, "Data"=w666, "Message"="Layout.Change", "Queue"=w674) -> ("error out"=w667:errorcluster, "Queue dup."=w671:refnum<queue>)  [unwired: 6 in]
      }
      event "Clock": Value Change {
        n239 = event-data() -> ("NewVal"=w677:u32)  [unwired: 1 in]
        n240 = To Variant(anything=w677) -> (Variant=w675:variant)
        n241 = call "Enqueue Message.vi"("Data"=w675, "Message"="DAC.Clock", "Queue"=w679) -> ("Queue dup."=w678:refnum<queue>)  [unwired: 7 in, 1 out]
      }
      event "Custom ADC / DAC": Value Change {
        n242 = event-data() -> ("NewVal"=w681:bool)  [unwired: 1 in]
        n243 = To Variant(anything=w681) -> (Variant=w680:variant)
        n244 = call "Enqueue Message.vi"("Data"=w680, "Message"="DAC.Switch", "Queue"=w684) -> ("Queue dup."=w683:refnum<queue>)  [unwired: 7 in, 1 out]
      }
      event Panel Close? {
        w689 = TRUE ("Rejeter ?")
        n245 = event-data() -> ()  [unwired: 1 in, 1 out]
        n246 = call "Enqueue Message.vi"("Prioritary message"=TRUE ("Message prioritaire ? (F)"), "Message"="Close", "Queue"=w688) -> ("error out"=w685:errorcluster, "Queue dup."=w686:refnum<queue>)  [unwired: 7 in]
        n247 = event-data ("Event Filter Node")("Discard?"=w689) -> ()  [unwired: 1 in, 1 out]
      }
      event User Event {
        n248 = event-data() -> ()  [unwired: 1 in, 1 out]
      }
    }
    n249 = case shown="Error" w642 {
      tunnel: [w647 TRUE ("Rejeter ?")] -> w644
      tunnel: w645 -> [w647 _]
      tunnel: w643 -> [_ w650]
      frame No Error {
      }
      frame Error {
        n250 = call "Enqueue Message.vi"("Prioritary message"=TRUE ("Message prioritaire ? (F)"), "Message"="Exit", "Queue"=w650) -> ()  [unwired: 7 in, 2 out]
      }
    }
  }
  n251 = Unregister For Events(event registration refnum=w5, error in=w6) -> (error out=w4:errorcluster)
  n252 = Merge Errors(w4, w12) -> (w8:errorcluster)
  n253 = flat-sequence {
    tunnel: w8 -> [w695]
    tunnel: w7 -> [w694]
    tunnel: [w693] -> w1
    tunnel: [w698] -> w2
    tunnel: w1 -> [w698]
    frame #0 {
      n254 = call "Destroy User Event - Stop.vi"("entrée d'erreur (pas d'erreur)"=w695, "Événement utilisateur - Arrêt"=w694) -> ("sortie d'erreur"=w696:errorcluster)  [unwired: 9 in]
      n255 = call <vilib>:"Simple Error Handler.vi"("error in (no error)"=w696) -> ("error out"=w693:errorcluster)  [unwired: 4 in, 4 out]
    }
    frame #1 {
      n256 = Request Deallocation(TRUE ("flag")) -> ()
    }
  }
  n257 = call <vilib>:"Clear Errors.vi"("error in (no error)"=w2) -> ()  [unwired: 5 in, 2 out]
